vi "InjectModel.vi"(8 "error in (no error)":errorcluster, 10 "Model":refnum<class "Model.lvclass">, 11 "Controller in":refnum<class "Controller.lvclass">) -> (0 "error out":errorcluster, 3 "Controller out":refnum<class "Controller.lvclass">)   [LabVIEW 2020, in "Page2.lvlib" / "Controller.lvclass"]
uses:
  Controller.lvclass
  Model/Model/Model.lvclass
  Controller.lvclass/Controller.ctl
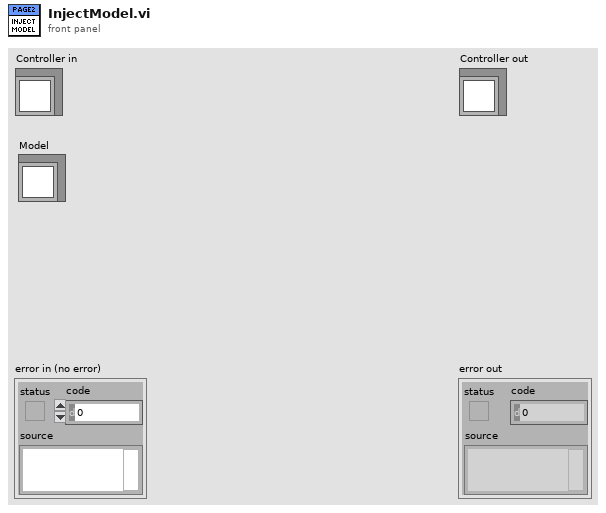
[diagram p1: front panel]
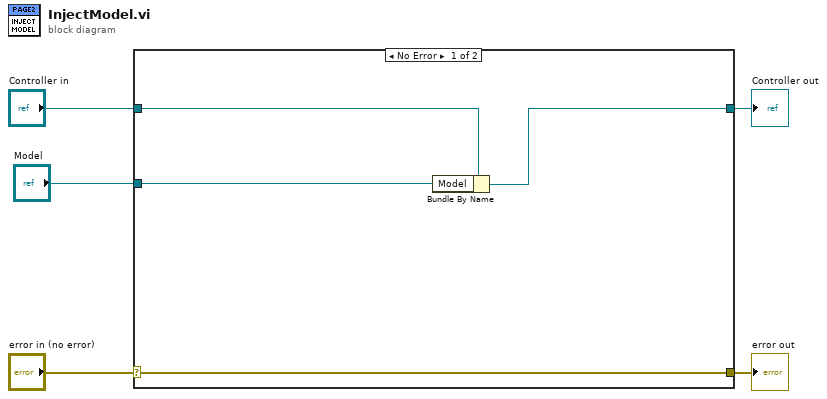
[diagram p0: block diagram]
diagram:
  n1 = case shown="No Error" "error in (no error)" {
    selector: "error in (no error)" -> [w9 w11]
    tunnel: [w9 w11] -> w4
    tunnel: [w6 w10] -> w2
    tunnel: "Controller in" -> [w8 w10]
    tunnel: "Model" -> [w7 _]
    frame No Error {
      n2 = Bundle By Name(cluster=w8, "Model"=w7) -> (w6:refnum<class "Controller.lvclass">)
    }
    frame Error {
    }
  }
  "error out" <- w4
  "Controller out" <- w2
